vi "Remove Boundary.vi"(1 "deleted pixel number":i32, 2 "input":dbl[][](array[numeric])) -> (0 "output":dbl[][](array[numeric]))   [LabVIEW 2014]
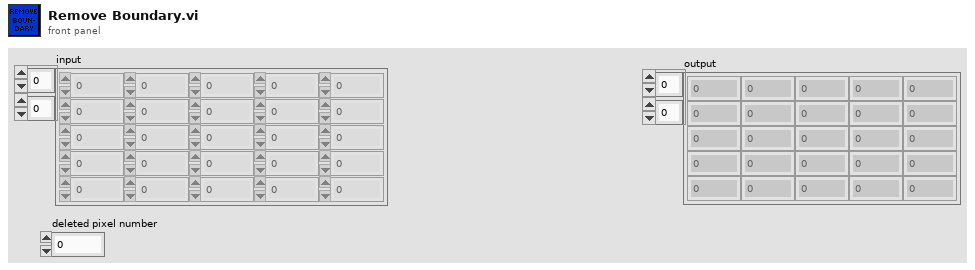
[diagram p1: front panel]
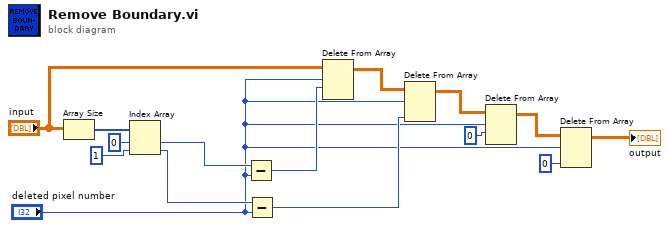
[diagram p0: block diagram]
diagram:
  n1 = Array Size(array="input") -> (size(s)=w15:i32[])
  n2 = Index Array(array=w15, index #1=0 ("index"), index #2=1 ("index")) -> (element #1=w11:i32, element #2=w10:i32)
  n3 = Subtract(x=w11, y="deleted pixel number") -> (x-y=w9:i32)
  n4 = Subtract(x=w10, y="deleted pixel number") -> (x-y=w8:i32)
  n5 = Delete From Array(array="input", length="deleted pixel number", index (row)=w9) -> (array with subset deleted=w6:dbl[][])  [unwired: 1 in, 1 out]
  n6 = Delete From Array(array=w6, length="deleted pixel number", index (col)=w8) -> (array with subset deleted=w7:dbl[][])  [unwired: 1 in, 1 out]
  n7 = Delete From Array(array=w7, length="deleted pixel number", index (row)=0) -> (array with subset deleted=w4:dbl[][])  [unwired: 1 in, 1 out]
  n8 = Delete From Array(array=w4, length="deleted pixel number", index (col)=0 ("disabled index (col)")) -> (array with subset deleted=→"output":dbl[][])  [unwired: 1 in, 1 out]
